vi "MDPtr ValidateFlattenToString2.vi"() -> ()   [LabVIEW 2017]
uses:
  <vilib>/Utility/High Resolution Relative Seconds.vi
panel:
  out "length 2":i32
  out "length":i32
  out "Waveform Graph 5":dbl[](graph)
  out "Waveform Graph 4":dbl[](graph)
  out "x-y 2":u32
  out "Waveform Graph 3":dbl[](graph)
  out "Waveform Graph 2":i32[](graph)
  out "Waveform Graph":dbl[](graph)
  out "x-y":u32
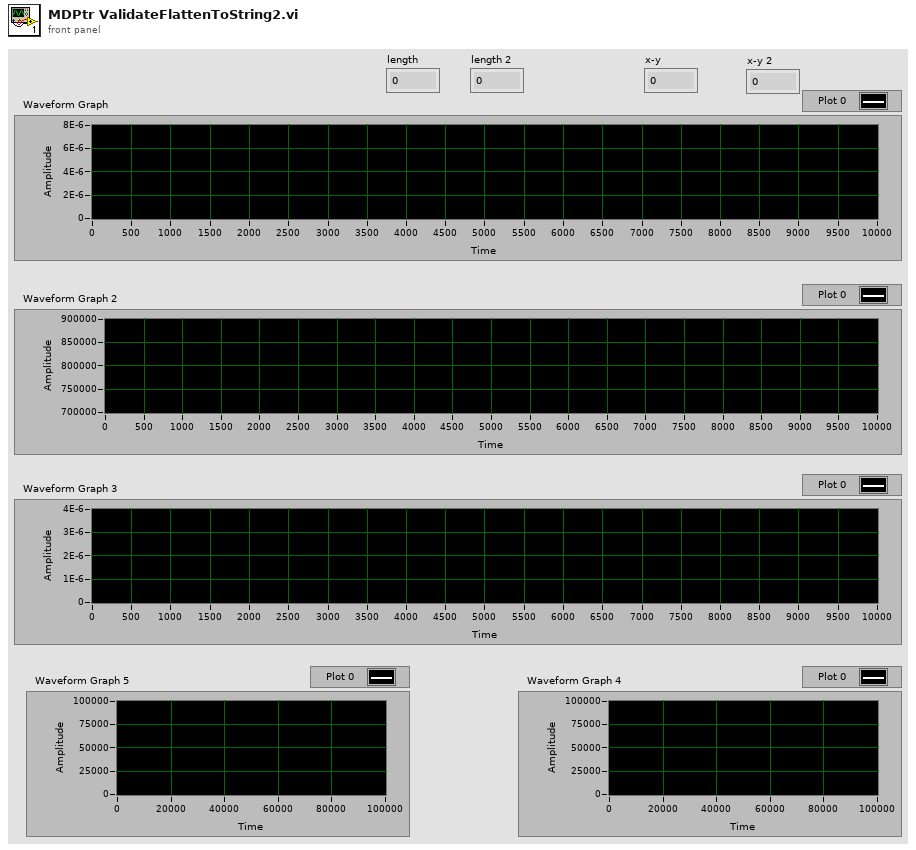
[diagram p1: front panel]
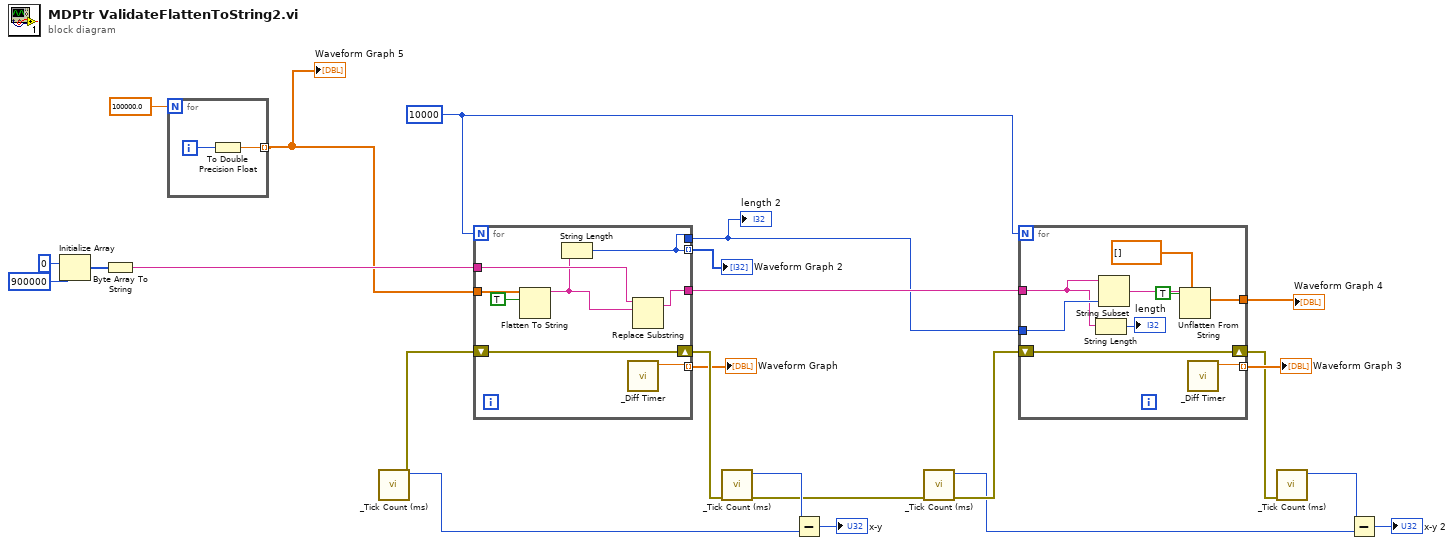
[diagram p0: block diagram]
diagram:
  w9 = 10000
  n1 = Initialize Array(u8 0 ("element"), 900000 ("dimension size")) -> (w6:u8[])
  n2 = Byte Array To String(unsigned byte array=w6) -> (string=w5:string)
  n3 = for {
    N: 100000.0 ("Fs") -> [_]
    tunnel: [w25] -> w2 mode=indexing
    i -> [w26]
    n4 = To Double Precision Float(number=w26) -> (double precision float=w25:dbl)
  }
  "Waveform Graph 5" <- w2
  n5 = call "_Tick Count (ms).vi"() -> ("error out"=w22:errorcluster, "millisecond timer value"=w23:u32)  [unwired: 10 in]
  n6 = for {
    N: w9 -> [_]
    tunnel: w2 -> [w34]
    tunnel: [w33] -> w19 mode=indexing
    shift-right: [w32] -> w21
    shift-left: w22 -> [w32]
    tunnel: [w28] -> w18 mode=indexing
    tunnel: [w29] -> w10
    tunnel: [w28] -> w4
    tunnel: w5 -> [w31]
    n7 = Flatten To String(anything=w34, prepend array or string size? (T)=TRUE) -> (data string=w30:string)  [unwired: 2 in, 2 out]
    n8 = String Length(string=w30) -> (length=w28:i32)
    n9 = call "_Diff Timer.vi"() -> ("time diff(s)"=w33:dbl)  [unwired: 10 in, 1 out]
    n10 = Replace Substring(4:w30, 5:w31) -> (1:w29:string)  [unwired: 2 in, 1 out]
  }
  "Waveform Graph" <- w19
  "Waveform Graph 2" <- w18
  "length 2" <- w4
  n11 = call "_Tick Count (ms).vi"("error in (no error)"=w21) -> ("error out"=w11:errorcluster, "millisecond timer value"=w24:u32)  [unwired: 9 in]
  n12 = Subtract(x=w24, y=w23) -> (x-y=→"x-y":u32)
  n13 = call "_Tick Count (ms).vi"("error in (no error)"=w11) -> ("error out"=w14:errorcluster, "millisecond timer value"=w13:u32)  [unwired: 9 in]
  n14 = for {
    N: w9 -> [_]
    tunnel: [w43] -> w17 mode=indexing
    shift-right: [w42] -> w15
    shift-left: w14 -> [w42]
    tunnel: w10 -> [w40]
    tunnel: w4 -> [w41]
    tunnel: [w36] -> w1
    n15 = String Length(string=w40) -> (length=→"length":i32)
    n16 = String Subset(string=w40, length (rest)=w41) -> (substring=w38:string)  [unwired: 1 in]
    n17 = Unflatten From String(type=dbl[] [] ("Fs"), binary string=w38, data includes array or string size? (T)=TRUE) -> (value=w36:dbl[])  [unwired: 2 in, 2 out]
    n18 = call "_Diff Timer.vi"() -> ("time diff(s)"=w43:dbl)  [unwired: 10 in, 1 out]
  }
  "Waveform Graph 3" <- w17
  "Waveform Graph 4" <- w1
  n19 = call "_Tick Count (ms).vi"("error in (no error)"=w15) -> ("millisecond timer value"=w12:u32)  [unwired: 9 in, 1 out]
  n20 = Subtract(x=w12, y=w13) -> (x-y=→"x-y 2":u32)
